vi "Configure Reference Oscillator.vi"(8 "error in (no error)":errorcluster, 10 "Reference Oscillator (Internal)":enum16{"Internal", "External"}(ring), 11 "SA-ESA in":refnum<class "SA-ESA.lvclass">) -> (0 "error out":errorcluster, 3 "SA-ESA out":refnum<class "SA-ESA.lvclass">)   [LabVIEW 2020, in "SA-ESA.lvclass"]
uses:
  SA-ESA.lvclass
  Spectrum Analyzer.lvclass
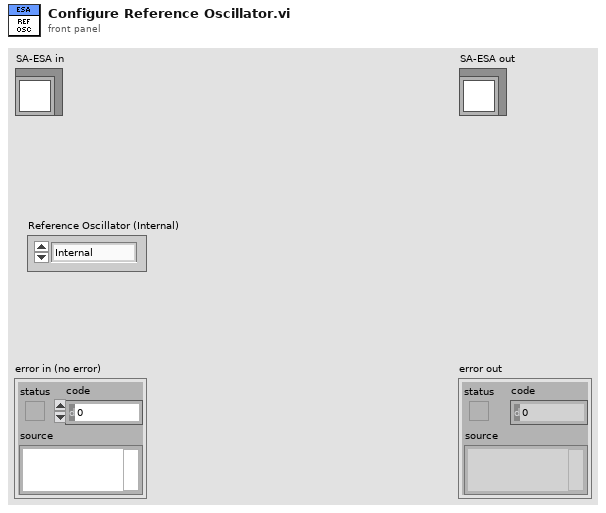
[diagram p1: front panel]
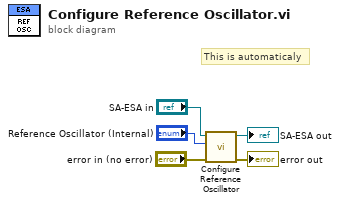
[diagram p0: block diagram]
diagram:
  # "This is automaticaly"
  n1 = call-parent "Configure Reference Oscillator.vi"("error in (no error)"="error in (no error)", "Reference Oscillator (Internal)"="Reference Oscillator (Internal)", "Spectrum Analyzer in"="SA-ESA in") -> ("error out"=→"error out":errorcluster, "Spectrum Analyzer out"=→"SA-ESA out":refnum<class "SA-ESA.lvclass">)  [unwired: 7 in]
